vi "Set Data Received.vi"(8 "error in (no error)":errorcluster caption="entrée d'erreur (pas d'erreur)", 10 "Data Received":bool, 11 "Server TCP_IP (Default) en entrée":refnum<class "Client TCP_IP (Default).lvclass">) -> (0 "error out":errorcluster caption="sortie d'erreur", 3 "Server TCP_IP (Default) en sortie":refnum<class "Client TCP_IP (Default).lvclass">)   [LabVIEW 2020, in "Library Instrument & Equipement.lvlib" / "Library TCP IP.lvlib" / "Client TCP_IP (Default).lvclass"]
uses:
  Client TCP_IP (Default).lvclass
  Client TCP_IP (Default).lvclass/Client TCP_IP (Default).ctl
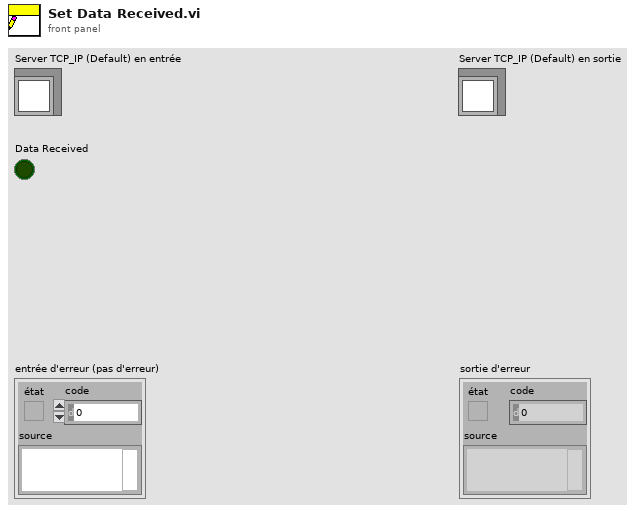
[diagram p1: front panel]
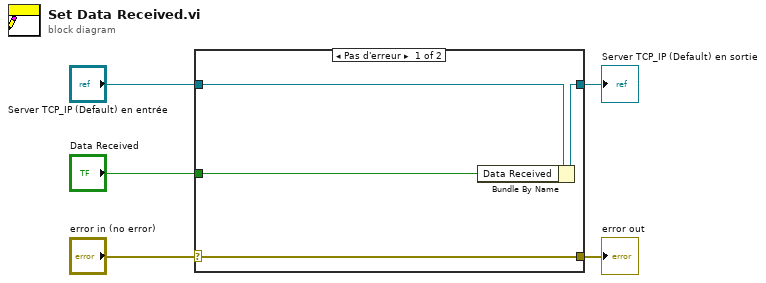
[diagram p0: block diagram]
diagram:
  n1 = case shown="Pas d'erreur" "error in (no error)" {
    selector: "error in (no error)" -> [w9 w10]
    tunnel: [w9 w10] -> w4
    tunnel: [w7 w11] -> w2
    tunnel: "Server TCP_IP (Default) en entrée" -> [w8 w11]
    tunnel: "Data Received" -> [w6 _]
    frame No Error {
      n2 = Bundle By Name(cluster=w8, "Data Received"=w6) -> (w7:refnum<class "Client TCP_IP (Default).lvclass">)
    }
    frame Error {
    }
  }
  "error out" <- w4
  "Server TCP_IP (Default) en sortie" <- w2
